vi "Simple XY Plot (SubVI).vi"(10 "y":dbl, 11 "x":dbl) -> (3 "Simple XY Position Plot":picture)   [LabVIEW 2017]
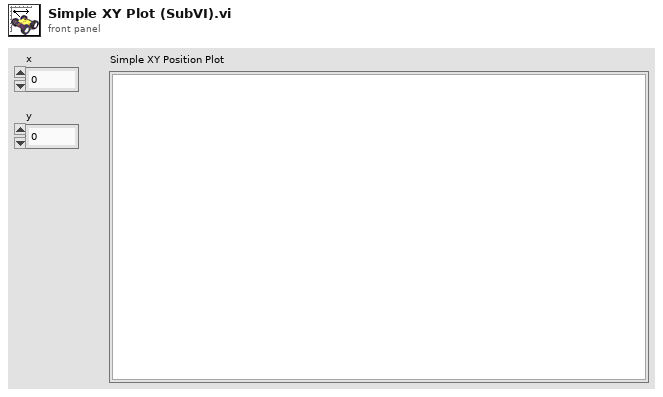
[diagram p1: front panel]
types:
  T1 = cluster{"Width":u16, "Style":enum32{"Solid", "Dash", "Dot", "DashDot", "DashDotDot"}}
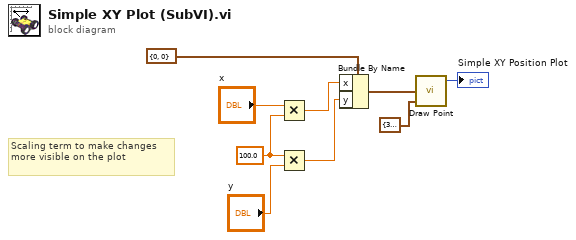
[diagram p0: block diagram]
diagram:
  w9 = 100.0 ("x")
  # "Scaling term to make changes more visible on the plot"
  n1 = Multiply(x="x", y=w9) -> (x*y=w7:dbl)
  n2 = Multiply(x=w9, y="y") -> (x*y=w8:dbl)
  n3 = Bundle By Name(cluster=cluster{"x":i16, "y":i16} {"x"=0, "y"=0} ("point(x,y)"), "x"=w7, "y"=w8) -> (w2:cluster{"x":i16, "y":i16})
  n4 = call <vilib>:"Draw Point.vi"("point(x,y)"=w2, "pen"=T1 {"Width"=3, "Style"=enum."Solid"}) -> ("new picture"=→"Simple XY Position Plot":picture)  [unwired: 7 in]
